vi "GetSWRevision.vi"(11 "File Path Control":path caption="File Path Control (leave blank to use Constants_Global value of EnFlo SW Folder)") -> (0 "This Folder's Last Changed Date":string, 1 "This Folder's Last Revision":string, 2 "LocalModifications":string, 3 "OverallRevision":string, 4 "standard error":string, 5 "standard output":string)   [LabVIEW 2016]
doc: "This VI uses the system's installed svn (subversion) software to return the revision number of the selected folder. Leaving the selected folder blank will use the global value of \"EnFlo SW Folder\".\nThe \"Overall Revision\" is the highest revision number in the entire hierarchy, recursing upwards as well as downwards- in other words, the revision which was checked out. The \"This Folder\" data is specific to the last changes to the selected folder."
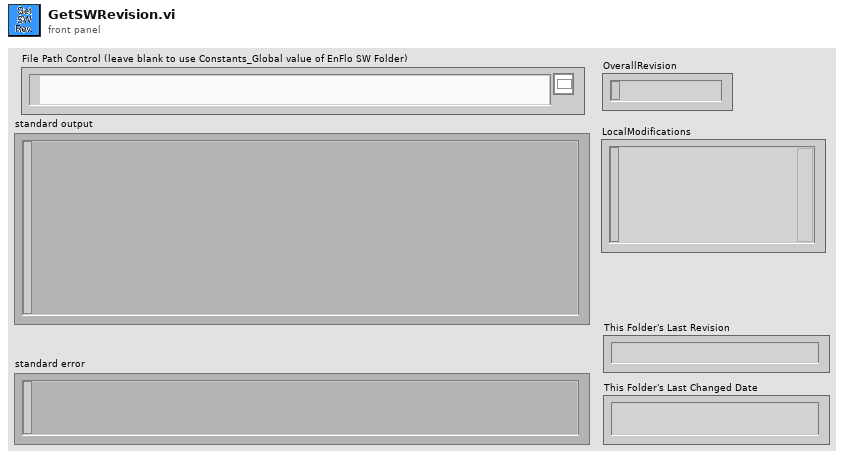
[diagram p1: front panel]
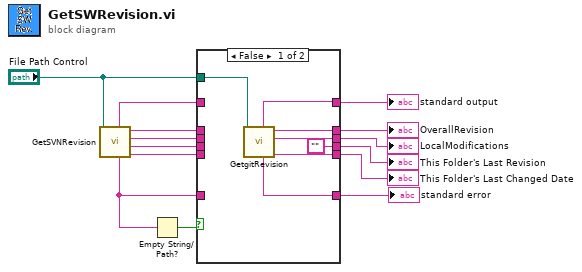
[diagram p0: block diagram]
diagram:
  n1 = call "GetSVNRevision.vi"("File Path Control"="File Path Control") -> ("This Folder's Last Changed Date"=w2:string, "This Folder's Last Revision"=w4:string, "LocalModifications"=w6:string, "OverallRevision"=w8:string, "standard error"=w10:string, "standard output"=w12:string)  [unwired: 5 in]
  n2 = Empty String/Path?(string/path=w10) -> (empty?=w14:bool)
  n3 = case shown="False" w14 {
    tunnel: [w21 w27] -> w13
    tunnel: w12 -> [_ w27]
    tunnel: [w17 w26] -> w11
    tunnel: w10 -> [_ w26]
    tunnel: [w20 w25] -> w9
    tunnel: w8 -> [_ w25]
    tunnel: [w19 w24] -> w7
    tunnel: w6 -> [_ w24]
    tunnel: ["" ("This Folder's Last Revision") w23] -> w5
    tunnel: w4 -> [_ w23]
    tunnel: [w18 w22] -> w3
    tunnel: w2 -> [_ w22]
    tunnel: "File Path Control" -> [w15 _]
    frame False {
      n4 = call "GetgitRevision.vi"("File Path Control"=w15) -> ("This Folder's Last Changed Date"=w18:string, "LocalModifications"=w19:string, "OverallRevision"=w20:string, "standard error"=w17:string, "standard output"=w21:string)  [unwired: 6 in]
    }
    frame True {
    }
  }
  "standard output" <- w13
  "standard error" <- w11
  "OverallRevision" <- w9
  "This Folder's Last Revision" <- w5
  "This Folder's Last Changed Date" <- w3
  "LocalModifications" <- w7
